vi "PowerGuardCreate.vi"(8 "error in":errorcluster) -> (0 "error out":errorcluster, 3 "Device Out":u64)   [LabVIEW 2012, in "Phidget Power Guard.lvlib"]
doc: "Creates a Phidget Temperature Sensor"
uses:
  <instrlib>/Phidgets/Phidget Power Guard/Phidget Power Guard.lvlib
  <instrlib>/Phidgets/Phidget Common/Phidget Common.lvlib
  phidget22.dll
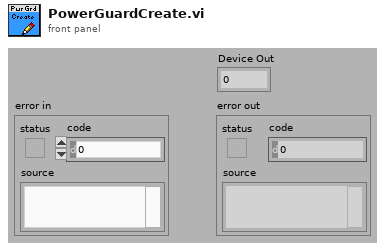
[diagram p1: front panel]
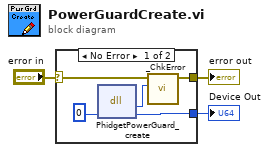
[diagram p0: block diagram]
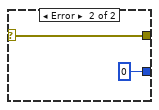
[diagram p2: hidden frame]
diagram:
  n1 = case shown="No Error" "error in" {
    selector: "error in" -> [w8 w10]
    tunnel: [w7 w10] -> w2
    tunnel: [w5 0 ("return type")] -> w1
    frame No Error {
      n2 = dll-call lib="phidget22.*" fn="PhidgetPowerGuard_create"("phid"=u64 0) -> ("return type"=w4:i32, "phid"=w5:u64)  [unwired: 3 in, 2 out]
      n3 = call <instrlib>:"_ChkError.vi"("Return Code"=w4, "error in (no error)"=w8) -> ("error out"=w7:errorcluster)  [unwired: 9 in]
    }
    frame Error {
    }
  }
  "error out" <- w2
  "Device Out" <- w1
